vi "WriteManyChannels.vi"() -> ()   [LabVIEW 2021]
uses:
  <vilib>/xnet/xnet.llb/XNET Frame CAN.ctl
  <vilib>/xnet/xnet.llb/XNET Frame Type CAN.ctl
  <vilib>/xnet/xnet.llb/XNET Create Session (Frame Output Stream).vi
  <vilib>/xnet/xnet.llb/XNET Write (Frame CAN).vi
  <resource>/objmgr/xnet.rc
panel:
  in  "milliseconds to wait":u32=1
  out "error out":errorcluster
  in  "stop":bool
  out "Num Frames":i32
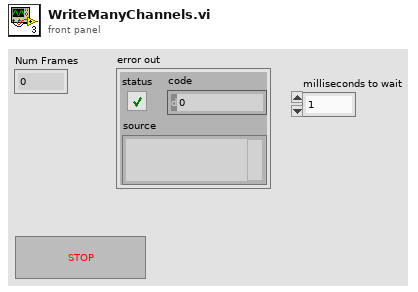
[diagram p1: front panel]
types:
  T1 = typedef "XNET Frame CAN.ctl" = cluster{"timestamp":timestamp, "payload":u8[], "identifier":u32, "type":T2, "extended?":bool, "echo?":bool}
  T2 = typedef "XNET Frame Type CAN.ctl" = u8
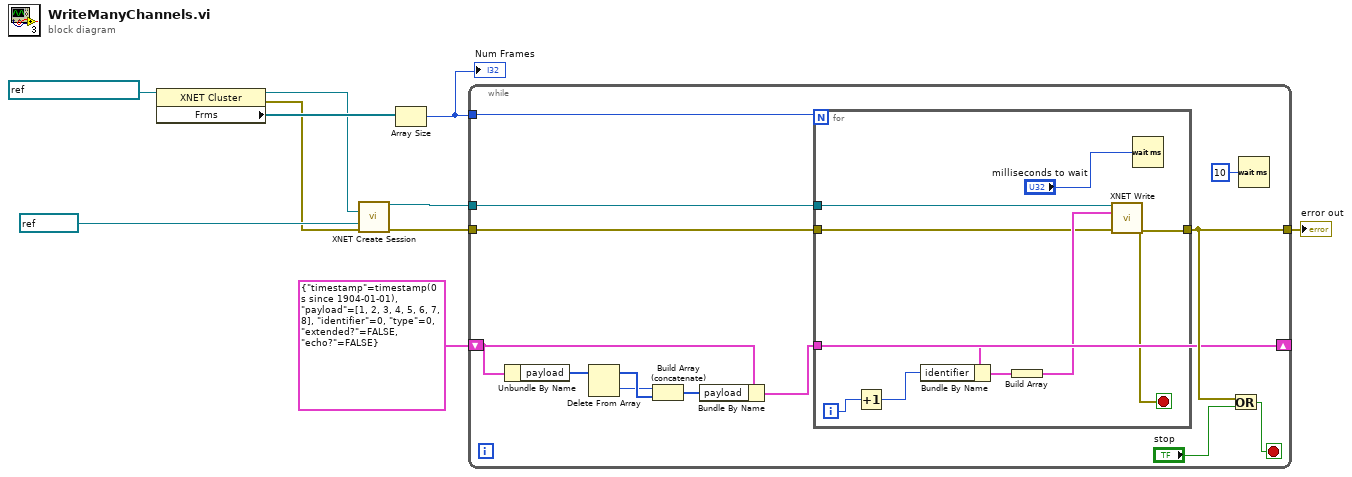
[diagram p0: block diagram]
diagram:
  n1 = property class="XNET Cluster"(reference=refnum<k21> "ManyXnetChannels" ("XNET Cluster")) -> (reference out=w2:refnum<k21>, error out=w3:errorcluster, "Frms"=w10:refnum<k21>[])  [unwired: 1 in]
  n2 = call-poly <vilib>:"XNET Create Session.vi"("cluster (:memory:)"=w2, "interface"=refnum<k21> "CAN2", "error in (no error)"=w3) -> ("session out"=w8:refnum<k21>, "error out"=w5:errorcluster)  [unwired: 11 in]
  n3 = Array Size(array=w10) -> (size(s)=w6:i32)
  "Num Frames" <- w6
  n4 = while {
    tunnel: w8 -> [w23]
    tunnel: w6 -> [w22]
    tunnel: w5 -> [w21]
    tunnel: [w18] -> w4
    shift-right: [w11] -> _
    shift-left: T1 {"timestamp"=timestamp(0 s since 1904-01-01), "payload"=[1, 2, 3, 4, 5, 6, 7, 8], "identifier"=0, "type"=0, "extended?"=FALSE, "echo?"=FALSE} ("CAN frame") -> [w16]
    stop <- w19 stop-if-true
    n5 = Unbundle By Name(w16) -> ("payload"=w15:u8[])
    n6 = Delete From Array(array=w15) -> (deleted portion=w12:u8, array with subset deleted=w14:u8[])  [unwired: 2 in]
    n7 = Build Array (concatenate)(w12, w14) -> (w13:u8[])
    n8 = Bundle By Name(cluster=w16, "payload"=w13) -> (w11:T1)
    n9 = for {
      N: w22 -> [_]
      tunnel: w23 -> [w32]
      tunnel: w11 -> [w31]
      tunnel: w21 -> [w26]
      tunnel: [w25] -> w18
      i -> [w28]
      stop <- w25 stop-if-true
      n10 = Increment(x=w28) -> (x+1=w27:i32)
      n11 = Bundle By Name(cluster=w31, "identifier"=w27) -> (w30:T1)
      n12 = Build Array(w30) -> (w29:T1[])
      n13 = call-poly <vilib>:"XNET Write.vi"("session in"=w32, "data"=w29, "error in (no error)"=w26) -> ("error out"=w25:errorcluster)  [unwired: 11 in, 1 out]
      n14 = Wait (ms)(milliseconds to wait="milliseconds to wait") -> ()  [unwired: 1 out]
    }
    n15 = Or(x=w18, y="stop") -> (x .or. y?=w19:bool)
    n16 = Wait (ms)(milliseconds to wait=u32 10) -> ()  [unwired: 1 out]
  }
  "error out" <- w4
